vi "Prepare Response.vi"(8 "error in (no error)":errorcluster, 11 "PUBREC in":refnum<class "PUBREC.lvclass">) -> (0 "error out":errorcluster, 1 "response prepared?":bool, 2 "ControlPacket response":refnum<class "ControlPacket.lvclass">, 3 "PUBREC out":refnum<class "PUBREC.lvclass">)   [LabVIEW 2013, in "PUBREC.lvclass"]
uses:
  PUBREC.lvclass
  ControlPacket/ControlPacket.lvclass
  ControlPacket/ControlPacket.lvclass/ControlPacket.ctl
  PUBREL/PUBREL.lvclass
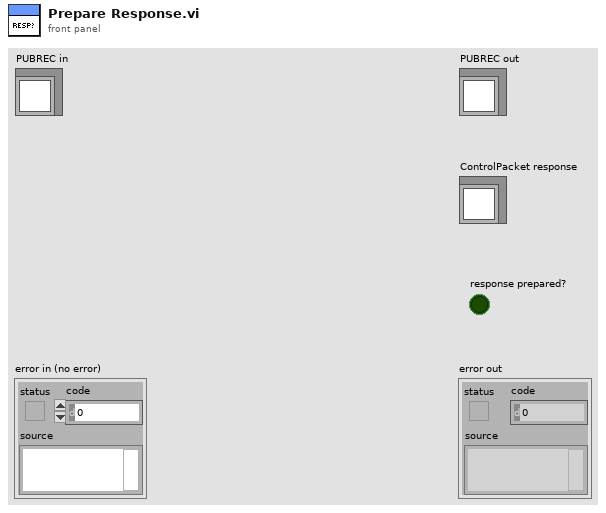
[diagram p1: front panel]
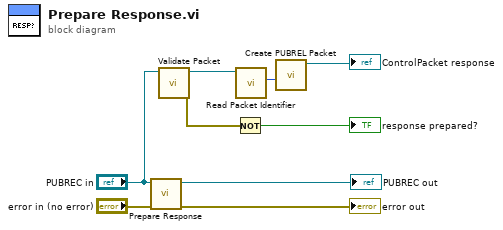
[diagram p0: block diagram]
diagram:
  n1 = call-parent "Prepare Response.vi"("error in (no error)"="error in (no error)", "ControlPacket in"="PUBREC in") -> ("error out"=→"error out":errorcluster, "ControlPacket out"=→"PUBREC out":refnum<class "PUBREC.lvclass">)  [unwired: 6 in, 2 out]
  n2 = call "Validate Packet.vi"("ControlPacket in"="PUBREC in") -> ("error out"=w2:errorcluster, "ControlPacket out"=w3:refnum<class "PUBREC.lvclass">)  [unwired: 9 in]
  n3 = Not(x=w2) -> (.not. x?=→"response prepared?":bool)
  n4 = call "Read Packet Identifier.vi"("ControlPacket in"=w3) -> ("Packet Identifier"=w6:u16)  [unwired: 9 in, 1 out]
  n5 = call "Create PUBREL Packet.vi"("Packet ID"=w6) -> ("PUBREL out"=→"ControlPacket response":refnum<class "PUBREL.lvclass">)  [unwired: 9 in, 1 out]
